vi "XYZ Stage-Cleanup.vi"(8 "error in (no error)":errorcluster, 10 "Z Stage config cluster":T1={"COM port"="COM7", "Baudrate"=0, "Type"=""}, 11 "XY Stage config cluster":T1={"COM port"="COM7", "Baudrate"=0, "Type"=""}) -> (0 "error out":errorcluster)   [LabVIEW 2020]
uses:
  Typedefs/XY Stage config cluster.ctl
  <vilib>/Utility/error.llb/DialogType.ctl
  Global Variables/General Globals.vi
  Drivers/Olympus IX BX Series/Olympus IX BX Series.lvlib
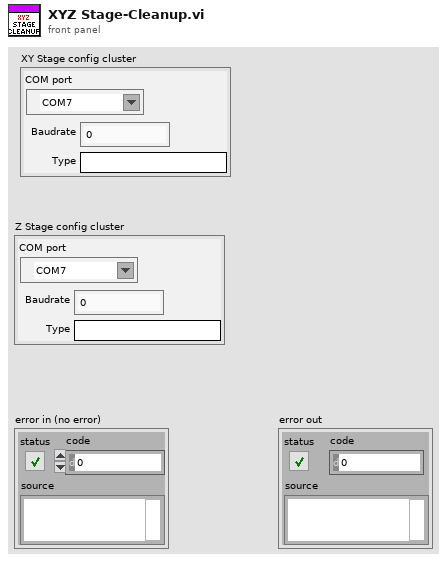
[diagram p1: front panel]
types:
  T1 = typedef "XY Stage config cluster.ctl" = cluster{"COM port":refnum<visa-resource-name>, "Baudrate":i32, "Type":string}
  T2 = typedef "DialogType.ctl" = u16
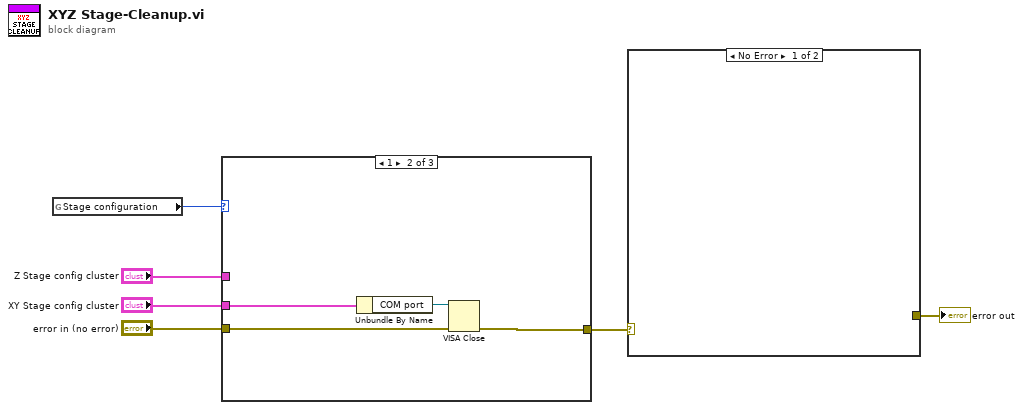
[diagram p0: block diagram]
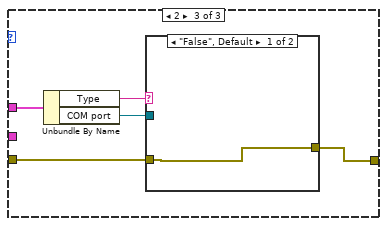
[diagram p3: hidden frame]
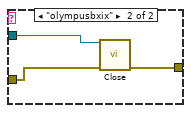
[diagram p4: hidden frame]
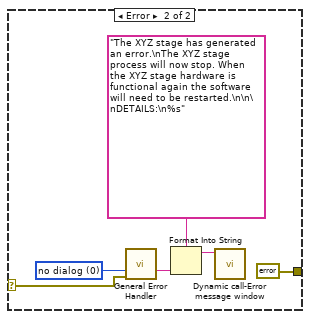
[diagram p5: hidden frame]
diagram:
  n1 = global read "General Globals.vi" "Stage configuration"() -> (w2:i32)
  n2 = case shown="1" w2 {
    tunnel: [w7 w11 w13] -> w6
    tunnel: "error in (no error)" -> [w7 w9 w14]
    tunnel: "XY Stage config cluster" -> [_ w8 _]
    tunnel: "Z Stage config cluster" -> [_ _ w16]
    frame 0, Default {
    }
    frame 1 {
      n3 = Unbundle By Name(w8) -> ("COM port"=w10:refnum<visa-resource-name>)
      n4 = VISA Close(VISA resource name=w10, error in (no error)=w9) -> (error out=w11:errorcluster)
    }
    frame 2 {
      n5 = Unbundle By Name(w16) -> ("Type"=w15:string, "COM port"=w12:refnum<visa-resource-name>)
      n6 = case shown="\"False\", Default" w15 {
        tunnel: w14 -> [w17 w20]
        tunnel: [w17 w19] -> w13
        tunnel: w12 -> [_ w18]
        frame "False", Default {
        }
        frame "olympusbxix" {
          n7 = call "Close.vi"("VISA Resource Name"=w18, "error in (no error)"=w20) -> ("error out"=w19:errorcluster)  [unwired: 13 in]
        }
      }
    }
  }
  n8 = case shown="No Error" w6 {
    selector: w6 -> [_ w22]
    tunnel: [_ errorcluster {"status"=FALSE, "code"=0, "source"=""} ("error out")] -> w4
    frame No Error {
    }
    frame Error {
      w24 = T2 0 items=["no dialog", "OK message", "continue or stop message", "OK message + warnings", "continue/stop + warnings"] ("type of dialog (OK msg:1)")
      n9 = call <vilib>:"General Error Handler.vi"("type of dialog (OK msg:1)"=w24, "error in (no error)"=w22) -> ("message"=w23:string)  [unwired: 9 in, 4 out]
      n10 = Format Into String(format string="The XYZ stage has generated an error.\nThe XYZ stage process will now stop. When the XYZ stage hardware is functional again the software will need to be restarted.\n\n\nDETAILS:\n%s" ("Error Source"), w23) -> (resulting string=w21:string)  [unwired: 2 in, 1 out]
      n11 = call "Dynamic call-Error message window.vi"("Error Message"=w21) -> ()  [unwired: 10 in, 1 out]
    }
  }
  "error out" <- w4
